vi "ParseVectorFile.SVG.GetObjects.vi"(8 "error in (no error)":errorcluster, 10 "Path":path, 11 "ParseVectorFile in":refnum<class "ParseVectorFile.lvclass">) -> (0 "error out":errorcluster, 3 "ParseVectorFile out":refnum<class "ParseVectorFile.lvclass">)   [LabVIEW 2019, in "ParseVectorFile.lvclass"]
uses:
  ParseVectorFile.lvclass
  ParseVectorFile.lvclass/ParseVectorFile.ctl
  ParseXML/ParseSVG.lvclass
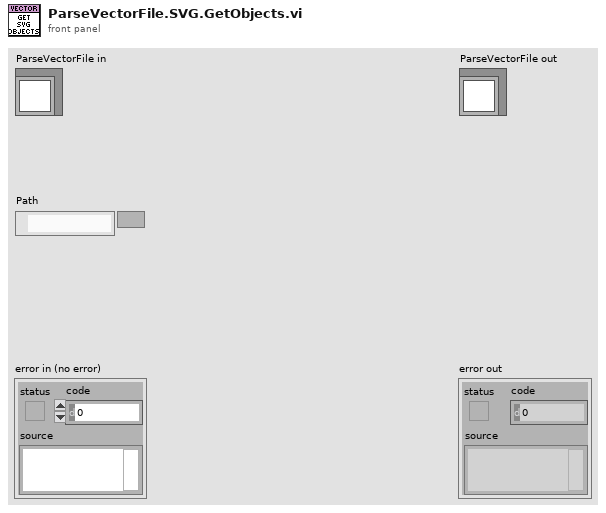
[diagram p1: front panel]
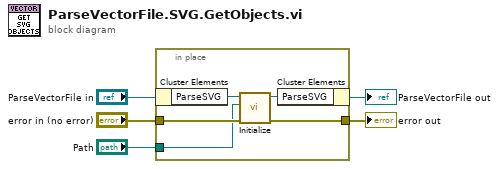
[diagram p0: block diagram]
diagram:
  n1 = in-place {
    in-place-border: "error in (no error)" -> [w8]
    in-place-border: [w7] -> w4
    in-place-border: "Path" -> [w6]
    n2 = in-place-cluster #1("ParseVectorFile in") -> ("ParseSVG"=w10:refnum<class "ParseSVG.lvclass">)
    n3 = call "Initialize.vi"("error in (no error)"=w8, "Path"=w6, "ParseXML in"=w10) -> ("error out"=w7:errorcluster, "ParseXML out"=w9:refnum<class "ParseSVG.lvclass">)  [unwired: 7 in]
    n4 = in-place-cluster #1("ParseSVG"=w9) -> (→"ParseVectorFile out":refnum<class "ParseVectorFile.lvclass">)
  }
  "error out" <- w4
